vi "Load Private Key and Certs.vi"() -> (0 "error out":errorcluster, 1 "Private Key":u8[](array[numeric]), 2 "Certificate Chain":cluster{"certificate":u8[]}[](array[cluster]))   [LabVIEW 2021, in "Secure Echo Broadcast Test Server Manager.lvlib"]
uses:
  Secure Echo Broadcast Test Server Manager.lvlib
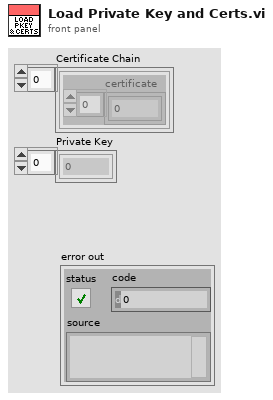
[diagram p1: front panel]
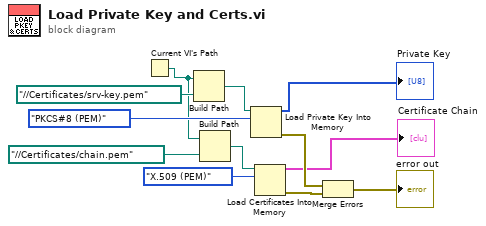
[diagram p0: block diagram]
diagram:
  n1 = Current VI's Path() -> (path=w6:path)
  n2 = Build Path(base path=w6, name or relative path=path "../../Certificates/srv-key.pem" ("key")) -> (appended path=w9:path)
  n3 = Build Path(base path=w6, name or relative path=path "../../Certificates/chain.pem" ("cert chain")) -> (appended path=w7:path)
  n4 = Load Private Key Into Memory(10:enum32{"PKCS#8 (PEM)", "PKCS#8 (DER)"}."PKCS#8 (PEM)" ("format"), 11:w9) -> (0:w5:errorcluster, 3:→"Private Key":u8[])  [unwired: 2 in]
  n5 = Load Certificates Into Memory(10:enum32{"X.509 (PEM)"}."X.509 (PEM)" ("format"), 11:w7) -> (0:w4:errorcluster, 3:→"Certificate Chain":cluster{"certificate":u8[]}[])  [unwired: 1 in]
  n6 = Merge Errors(w5, w4) -> (→"error out":errorcluster)
